vi "CRYExcel Manipulate.vi"(7 "sAction":string, 8 "error in (no error)":errorcluster, 9 "nData":i32, 10 "sData":string, 11 "report in":refnum<class "NI_report.lvclass">) -> (0 "error out":errorcluster, 1 "sData out":string[](array[string]), 2 "nData out":i32[](array[numeric]), 3 "report out":refnum<class "NI_report.lvclass">)   [LabVIEW 2013]
uses:
  <vilib>/Utility/NIReport.llb/NI_report.lvclass
  <vilib>/Utility/NIReport.llb/Excel/NI_Excel.lvclass
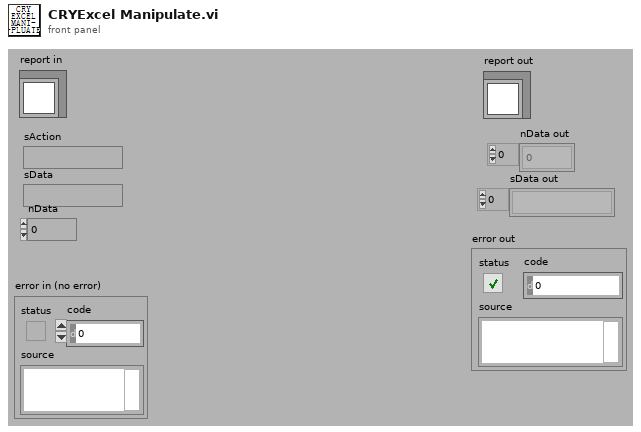
[diagram p1: front panel]
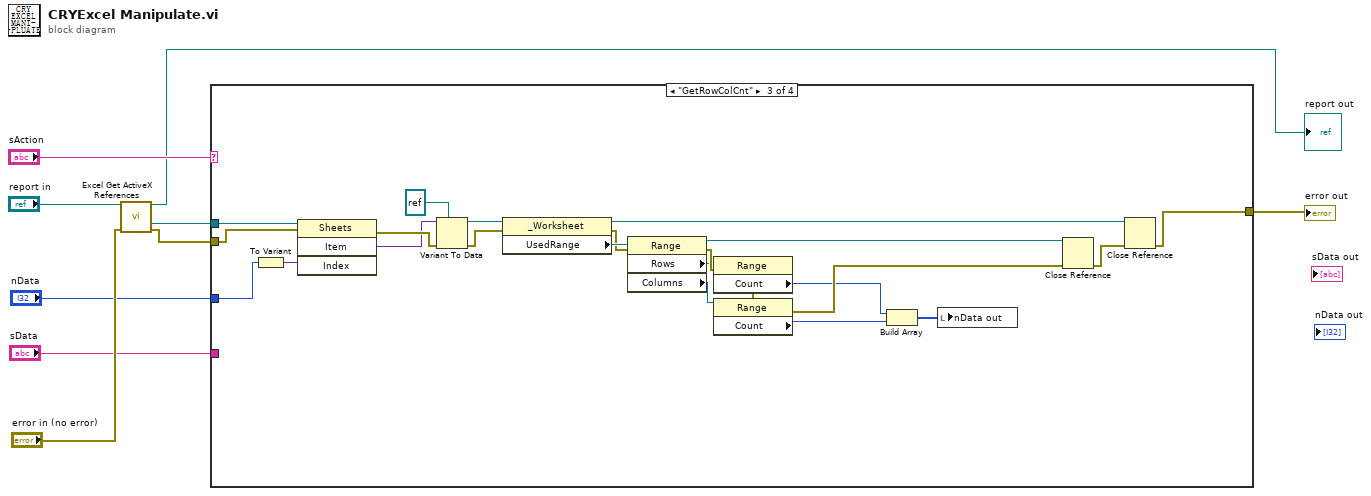
[diagram p0: block diagram]
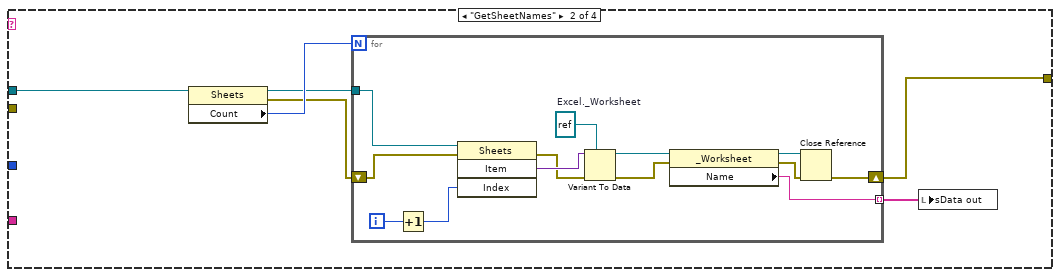
[diagram p3: hidden frame]
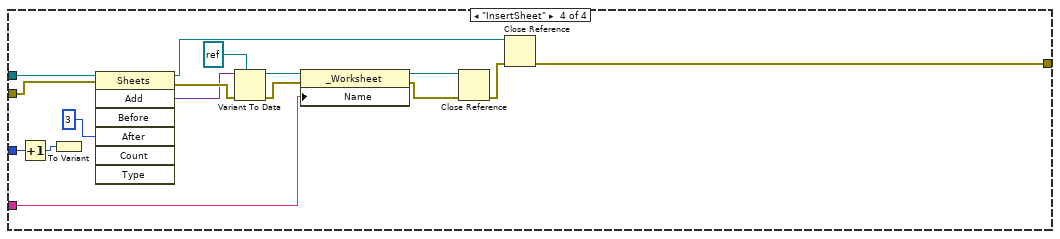
[diagram p4: hidden frame]
diagram:
  n1 = call <vilib>:"Excel Get ActiveX References.vi"("report in"="report in", "error in (no error)"="error in (no error)") -> ("report out"=→"report out":refnum<class "NI_report.lvclass">, "Excel.Sheets"=w3:refnum<k7>, "error out"=w6:errorcluster)  [unwired: 7 in, 4 out]
  n2 = case shown="\"GetRowColCnt\"" "sAction" {
    tunnel: w6 -> [_ _ w40 w62]
    tunnel: [_ w10 w29 w56] -> w4
    tunnel: w3 -> [_ w12 w41 w63]
    tunnel: "nData" -> [_ _ w34 w59]
    tunnel: "sData" -> [_ _ _ w55]
    frame Default {
    }
    frame "GetSheetNames" {
      n3 = property class="Sheets"(reference=w12) -> (reference out=w11:refnum<k7>, error out=w14:errorcluster, "Count"=w15:i32)  [unwired: 1 in]
      n4 = for {
        N: w15 -> [_]
        tunnel: w11 -> [w26]
        shift-right: [w23] -> w10
        shift-left: w14 -> [w22]
        tunnel: [w16] -> w13 mode=indexing
        i -> [w28]
        w21 = refnum<k7> refnum  # Excel._Worksheet
        n5 = Increment(x=w28) -> (x+1=w27:i32)
        n6 = invoke class="Sheets" method="Item"(reference=w26, error in=w22, "Index"=w27) -> (error out=w24:errorcluster, "Item"=w25:variant)  [unwired: 1 in, 2 out]
        n7 = Variant To Data(error in=w24, type=w21, Variant=w25) -> (data=w20:refnum<k7>, error out=w19:errorcluster)
        n8 = property class="_Worksheet"(reference=w20, error in=w19) -> (reference out=w17:refnum<k7>, error out=w18:errorcluster, "Name"=w16:string)
        n9 = Close Reference(reference=w17, error in (no error)=w18) -> (error out=w23:errorcluster)
      }
      n10 = local write "sData out"(w13) -> ()
    }
    frame "GetRowColCnt" {
      n11 = To Variant(anything=w34) -> (Variant=w48:variant)
      n12 = invoke class="Sheets" method="Item"(reference=w41, error in=w40, "Index"=w48) -> (error out=w51:errorcluster, "Item"=w50:variant)  [unwired: 1 in, 2 out]
      n13 = Variant To Data(error in=w51, type=refnum<k7> refnum ("Worksheets"), Variant=w50) -> (data=w42:refnum<k7>, error out=w35:errorcluster)
      n14 = property class="_Worksheet"(reference=w42, error in=w35) -> (reference out=w39:refnum<k7>, error out=w33:errorcluster, "UsedRange"=w44:refnum<k7>)
      n15 = property class="Range"(reference=w44, error in=w33) -> (reference out=w38:refnum<k7>, error out=w45:errorcluster, "Rows"=w43:refnum<k7>, "Columns"=w46:refnum<k7>)
      n16 = property class="Range"(reference=w43, error in=w45) -> (error out=w47:errorcluster, "Count"=w32:i32)  [unwired: 1 out]
      n17 = property class="Range"(reference=w46, error in=w47) -> (error out=w36:errorcluster, "Count"=w31:i32)  [unwired: 1 out]
      n18 = Build Array(w32, w31) -> (w30:i32[])
      n19 = local write "nData out"(w30) -> ()
      n20 = Close Reference(reference=w38, error in (no error)=w36) -> (error out=w37:errorcluster)
      n21 = Close Reference(reference=w39, error in (no error)=w37) -> (error out=w29:errorcluster)
    }
    frame "InsertSheet" {
      n22 = Increment(x=w59) -> (x+1=w53:i32)
      n23 = To Variant(anything=w53) -> ()  [unwired: 1 out]
      n24 = invoke class="Sheets" method="Add"(reference=w63, error in=w62, "After"=3 ("x+1")) -> (reference out=w58:refnum<k7>, error out=w67:errorcluster, "Add"=w66:variant)  [unwired: 4 in, 4 out]
      n25 = Variant To Data(error in=w67, type=refnum<k7> refnum ("Worksheets"), Variant=w66) -> (data=w64:refnum<k7>, error out=w60:errorcluster)
      n26 = property class="_Worksheet"(reference=w64, error in=w60, "Name"=w55) -> (reference out=w61:refnum<k7>, error out=w54:errorcluster)
      n27 = Close Reference(reference=w61, error in (no error)=w54) -> (error out=w57:errorcluster)
      n28 = Close Reference(reference=w58, error in (no error)=w57) -> (error out=w56:errorcluster)
    }
  }
  "error out" <- w4
